vi "GDSProject_GetAllClasses.vi"(1 "AnyProjectItemRefnum":refnum<vi>, 2 "TreeControlRef":refnum<vi>, 3 "ClassProviderName":string, 4 "RootParentTag":string="LabVIEW Object", 5 "error In":errorcluster) -> (15 "ClassPaths":path[](array[path]), 16 "ClassTags":string[](array[string]), 19 "error out":errorcluster)   [LabVIEW 2012]
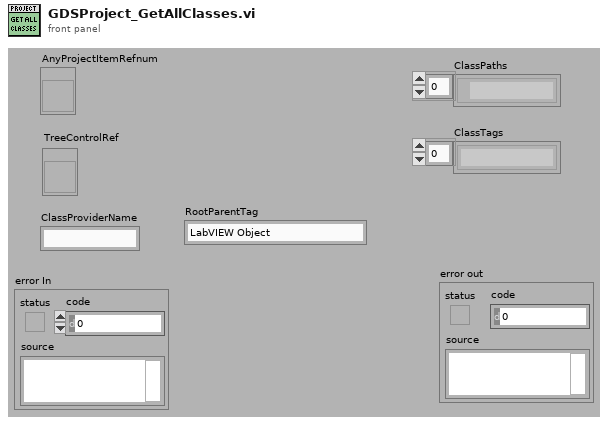
[diagram p1: front panel]
types:
  T1 = cluster{"Classes":refnum<vi>[], "Parents":refnum<vi>[], "ClassIneritance":cluster{string[]}[], "ClassTags":string[], "ClassPaths":path[], "ClassNames":string[]}
  T2 = typedef "GDSLvCLass_ClassSettingsType.ctl" = cluster{"ClassProviderName":string, "ClassTemplateUsed":string, "ClassTemplateVersion":string, "ClassDescription":string, "PlugIns":T3[], "ConnectorPanePattern":string}
  T3 = typedef "GDSLvClass_PlugIn.ctl" = cluster{"Type":T4, "ID":string, "Version":string, "Path":path, "Name":string, "Data":variant}
  T4 = typedef "GDSLvClass_PlugInTypes.ctl" = enum16{"DesignPattern", "MethodTypes"}
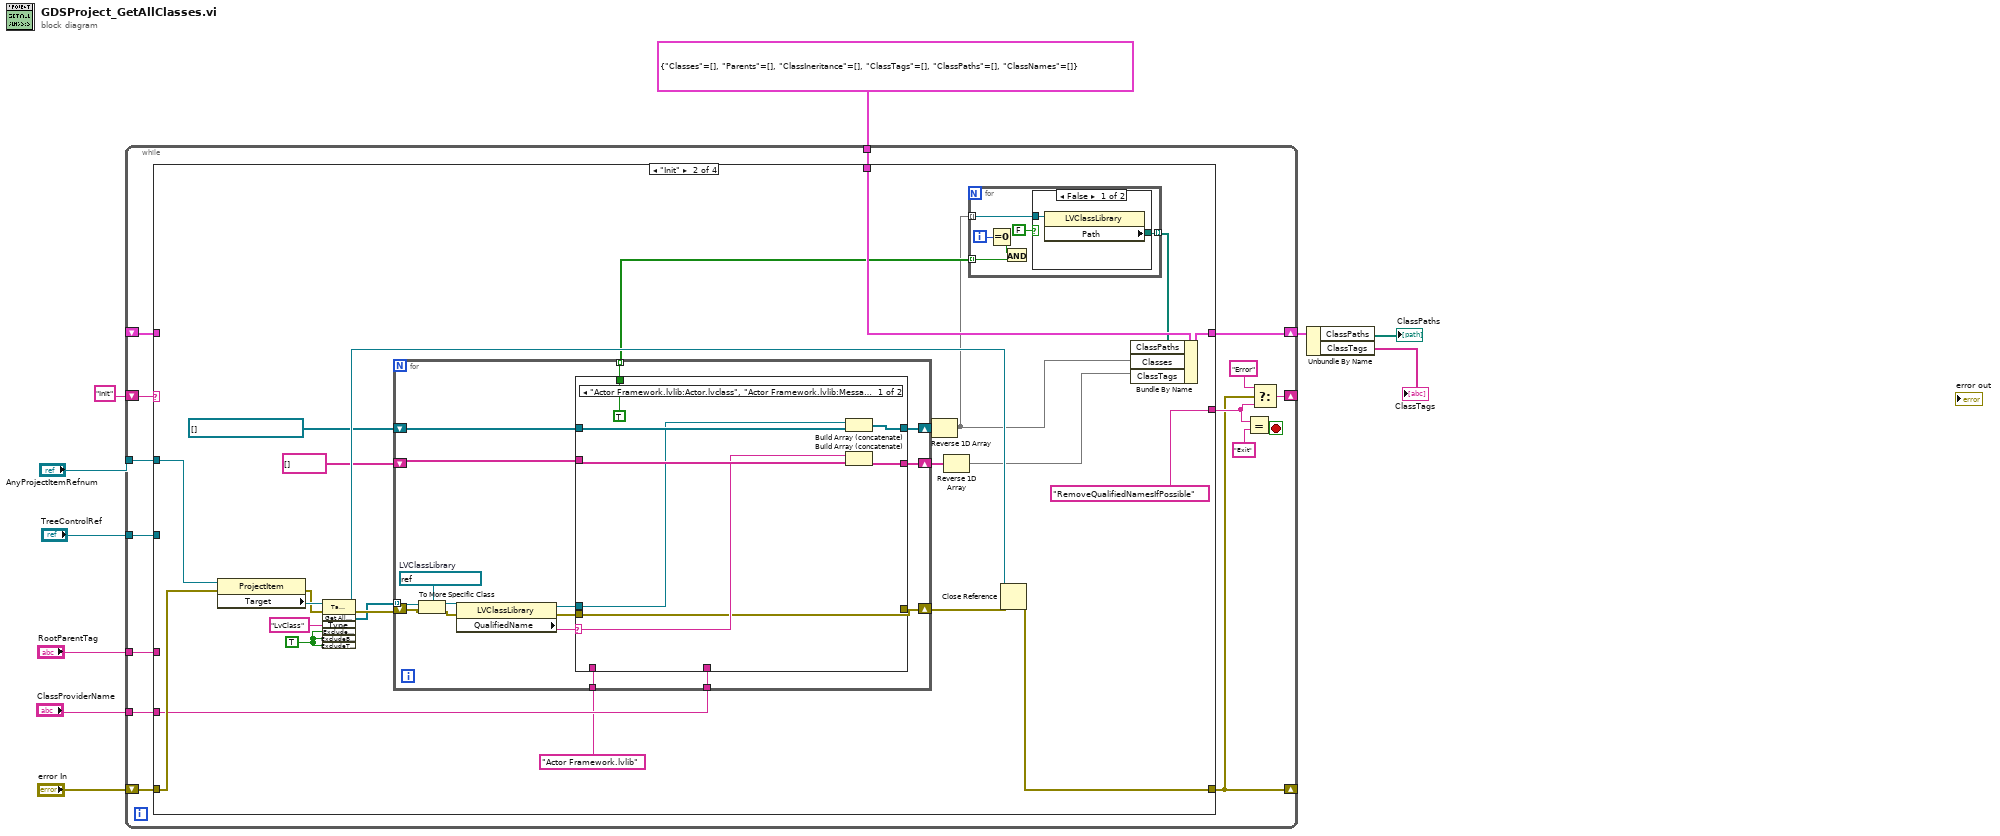
[diagram p0: block diagram]
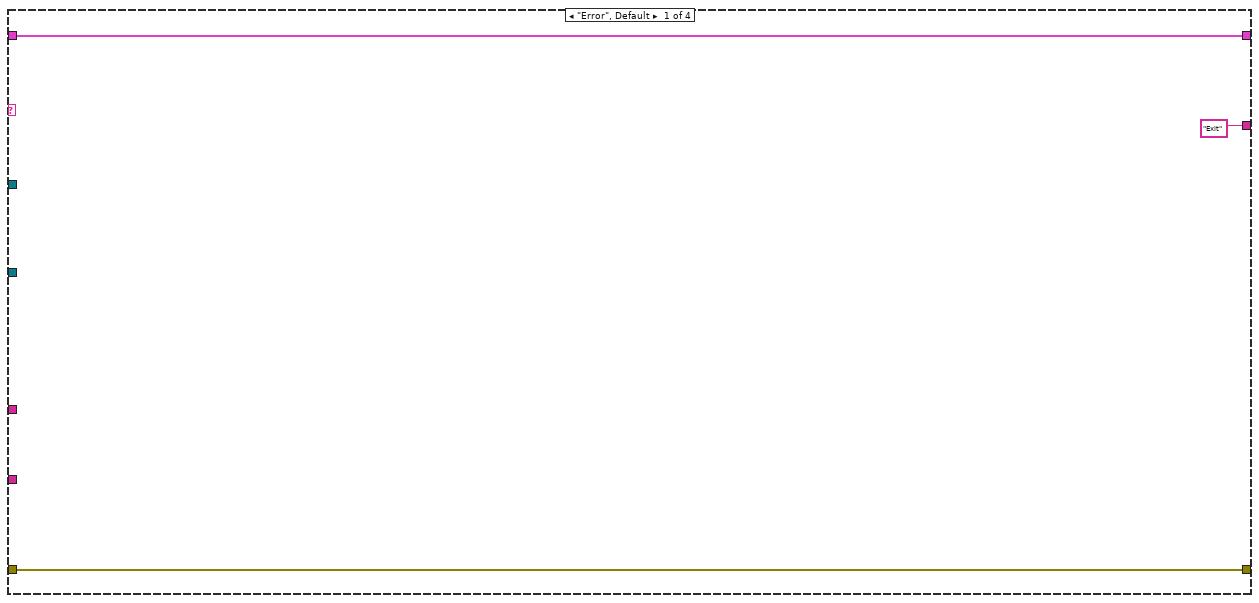
[diagram p2: hidden frame]
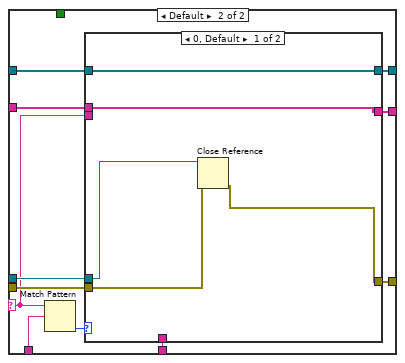
[diagram p4: hidden frame]
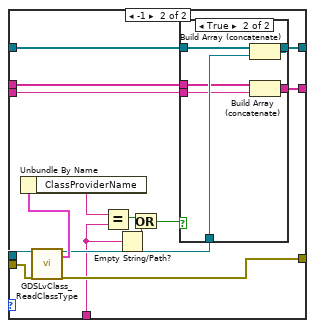
[diagram p5: hidden frame]
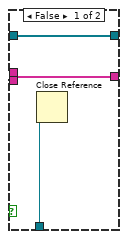
[diagram p6: hidden frame]
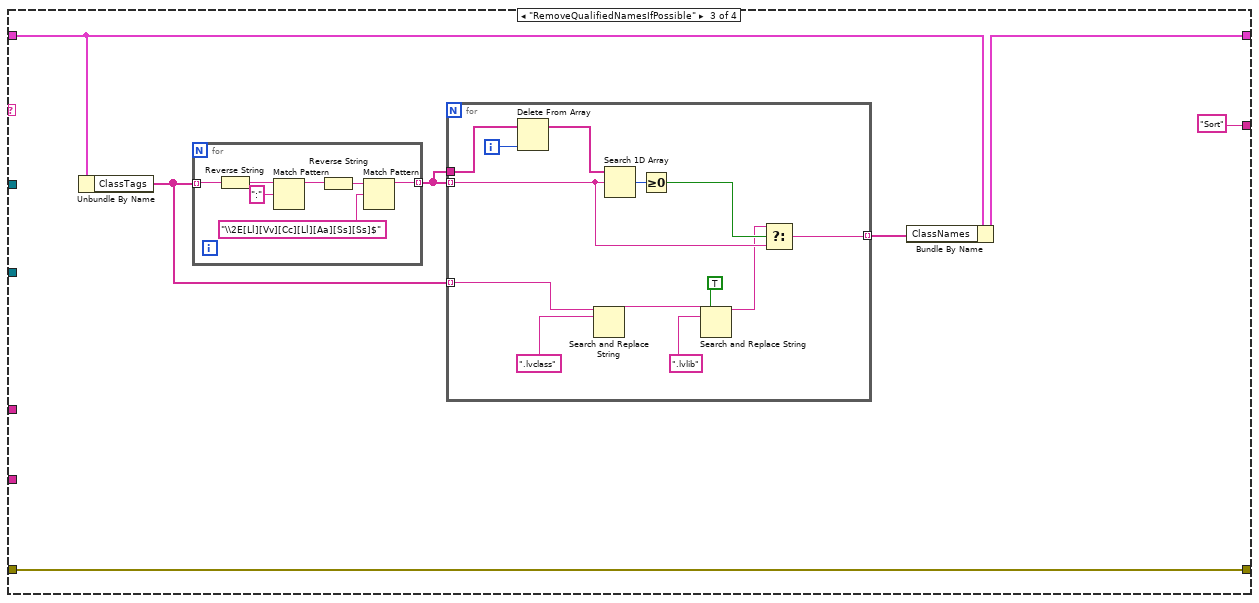
[diagram p7: hidden frame]
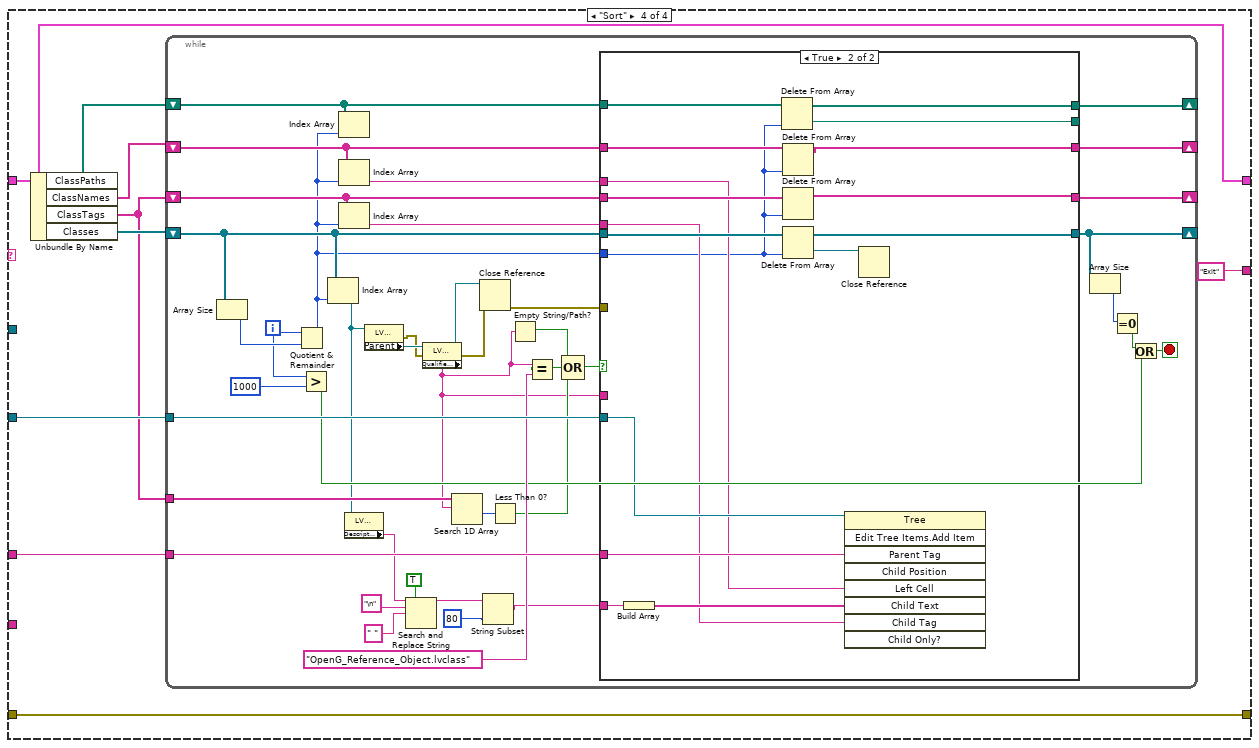
[diagram p8: hidden frame]
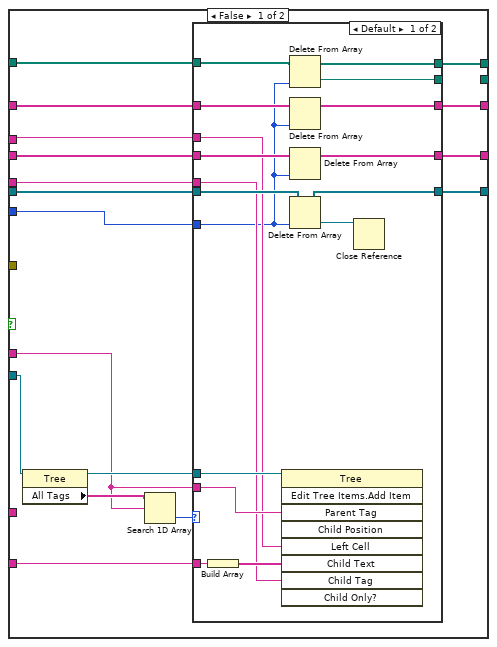
[diagram p9: hidden frame]
diagram:
  n1 = while {
    shift-right: [w18] -> _
    shift-left: "error In" -> [w25]
    shift-right: [w23] -> _
    shift-left: "Init" -> [w24]
    shift-right: [w17] -> w3
    shift-left: _ -> [w16]
    tunnel: "AnyProjectItemRefnum" -> [w15]
    tunnel: T1 {"Classes"=[], "Parents"=[], "ClassIneritance"=[], "ClassTags"=[], "ClassPaths"=[], "ClassNames"=[]} -> [w14]
    tunnel: "ClassProviderName" -> [w13]
    tunnel: "TreeControlRef" -> [w12]
    tunnel: "RootParentTag" -> [w11]
    stop <- w22 stop-if-true
    n2 = case shown="\"Init\"" w24 {
      tunnel: w25 -> [w28 w46 w125 w157]
      tunnel: [w28 w45 w125 w157] -> w18
      tunnel: ["Exit" "RemoveQualifiedNamesIfPossible" "Sort" "Exit"] -> w19
      tunnel: [w26 w43 w127 w155] -> w17
      tunnel: w16 -> [w26 _ w129 w155]
      tunnel: w15 -> [_ w48 _ _]
      tunnel: w14 -> [_ w44 _ _]
      tunnel: w13 -> [_ w42 _ _]
      tunnel: w12 -> [_ _ _ w156]
      tunnel: w11 -> [_ _ _ w158]
      frame "Error", Default {
      }
      frame "Init" {
        w50 = TRUE ("ExcludeDependencies")
        n3 = property class="ProjectItem"(reference=w48, error in=w46) -> (error out=w35:errorcluster, "Target"=w36:refnum<vi>)  [unwired: 1 out]
        n4 = invoke class="TargetItem" method="Get All Descendents"(reference=w36, error in=w35, "Type"="LvClass", "Exclude Dependencies"=w50, "ExcludeBuilds"=w50, "ExcludeTargets"=w50) -> (reference out=w49:refnum<vi>, error out=w47:errorcluster, "All Descendents"=w33:refnum<vi>[])  [unwired: 1 in, 4 out]
        n5 = for {
          tunnel: w33 -> [w76] mode=indexing
          shift-right: [w61] -> w38
          shift-left: refnum<vi>[] [] -> [w74]
          shift-right: [w72] -> w34
          shift-left: w47 -> [w73]
          tunnel: w42 -> [w71]
          shift-right: [w70] -> w39
          shift-left: string[] [] -> [w69]
          tunnel: [w63] -> w32 mode=indexing
          tunnel: "Actor Framework.lvlib" ("Type") -> [w62]
          w75 = refnum<vi> refnum  # LVClassLibrary
          n6 = To More Specific Class(target class=w75, reference=w76, error in=w73) -> (specific class reference=w68:refnum<vi>, error out=w66:errorcluster)
          n7 = property class="LVClassLibrary"(reference=w68, error in=w66) -> (reference out=w67:refnum<vi>, error out=w65:errorcluster, "QualifiedName"=w64:string)
          n8 = case shown="\"Actor Framework.lvlib:Actor.lvclass\", \"Actor Framework.lvlib:Message.lvclass\"" w64 {
            selector: w64 -> [w80 w85]
            tunnel: [w84 w86] -> w61
            tunnel: w74 -> [w78 w95]
            tunnel: [w79 w94] -> w72
            tunnel: w71 -> [_ w93]
            tunnel: [w83 w92] -> w70
            tunnel: w69 -> [w82 w91]
            tunnel: w67 -> [w77 w90]
            tunnel: w65 -> [w79 w89]
            tunnel: [TRUE _] -> w63
            tunnel: w62 -> [_ w88]
            frame "Actor Framework.lvlib:Actor.lvclass", "Actor Framework.lvlib:Message.lvclass" {
              n9 = Build Array (concatenate)(w77, w78) -> (w84:refnum<vi>[])
              n10 = Build Array (concatenate)(w80, w82) -> (w83:string[])
            }
            frame Default {
              n11 = Match Pattern(string=w85, regular expression=w88) -> (offset past match=w87:i32)  [unwired: 1 in, 3 out]
              n12 = case shown="0, Default" w87 {
                tunnel: [w100 w115] -> w86
                tunnel: w95 -> [w100 w114]
                tunnel: [w96 w111] -> w94
                tunnel: w93 -> [_ w109]
                tunnel: [w99 w105] -> w92
                tunnel: w91 -> [w99 w104]
                tunnel: w90 -> [w98 w103]
                tunnel: w89 -> [w97 w102]
                tunnel: w85 -> [_ w101]
                frame 0, Default {
                  n13 = Close Reference(reference=w98, error in (no error)=w97) -> (error out=w96:errorcluster)
                }
                frame -1 {
                  n14 = call <resource>:"GDSLvClass_ReadClassType.vi"("Class Refnum In"=w103, "error in (no error)"=w102) -> ("Class Refnum Out"=w112:refnum<vi>, "ClassSettings"=w113:T2, "error out"=w111:errorcluster)  [unwired: 15 in]
                  n15 = Unbundle By Name(w113) -> ("ClassProviderName"=w110:string)
                  n16 = Equal?(x=w110, y=w109) -> (x = y?=w108:bool)
                  n17 = Empty String/Path?(string/path=w109) -> (empty?=w107:bool)
                  n18 = Or(x=w108, y=w107) -> (x .or. y?=w106:bool)
                  n19 = case shown="True" w106 {
                    tunnel: [w118 w124] -> w115
                    tunnel: w114 -> [w118 w123]
                    tunnel: w112 -> [w117 w122]
                    tunnel: [w116 w121] -> w105
                    tunnel: w104 -> [w116 w120]
                    tunnel: w101 -> [_ w119]
                    frame False {
                      n20 = Close Reference(reference=w117) -> ()  [unwired: 1 in, 1 out]
                    }
                    frame True {
                      n21 = Build Array (concatenate)(w123, w122) -> (w124:refnum<vi>[])
                      n22 = Build Array (concatenate)(w120, w119) -> (w121:string[])
                    }
                  }
                }
              }
            }
          }
        }
        n23 = Reverse 1D Array(array=w38) -> (reversed array=w31:refnum<vi>[])
        n24 = Reverse 1D Array(array=w39) -> (reversed array=w30:string[])
        n25 = for {
          tunnel: w31 -> [w58] mode=indexing
          tunnel: [w57] -> w37 mode=indexing
          tunnel: w32 -> [w54] mode=indexing
          i -> [w56]
          n26 = Equal To 0?(x=w56) -> (x = 0?=w55:bool)
          n27 = And(x=w55, y=w54) -> ()  [unwired: 1 out]
          n28 = case shown="False" FALSE {
            tunnel: w58 -> [w60 _]
            tunnel: [w59 _] -> w57
            frame False {
              n29 = property class="LVClassLibrary"(reference=w60) -> ("Path"=w59:path)  [unwired: 1 in, 2 out]
            }
            frame True {
            }
          }
        }
        n30 = Close Reference(reference=w49, error in (no error)=w34) -> (error out=w45:errorcluster)
        n31 = Bundle By Name(cluster=w44, "ClassPaths"=w37, "Classes"=w31, "ClassTags"=w30) -> (w43:T1)
      }
      frame "RemoveQualifiedNamesIfPossible" {
        n32 = Unbundle By Name(w129) -> ("ClassTags"=w130:string[])
        n33 = for {
          tunnel: w130 -> [w151] mode=indexing
          tunnel: [w145] -> w131 mode=indexing
          n34 = Reverse String(1:w151) -> (0:w150:string)
          n35 = Match Pattern(string=w150, regular expression=":") -> (before substring=w148:string)  [unwired: 1 in, 3 out]
          n36 = Reverse String(1:w148) -> (0:w146:string)
          n37 = Match Pattern(string=w146, regular expression="\\2E[Ll][Vv][Cc][Ll][Aa][Ss][Ss]$") -> (before substring=w145:string)  [unwired: 1 in, 3 out]
        }
        n38 = for {
          tunnel: w131 -> [w142] mode=indexing
          tunnel: w131 -> [w140]
          tunnel: w130 -> [w133] mode=indexing
          tunnel: [w141] -> w128 mode=indexing
          i -> [w138]
          n39 = Delete From Array(array=w140, index=w138) -> (array with subset deleted=w139:string[])  [unwired: 1 in, 1 out]
          n40 = Search and Replace String(input string=w133, search string=".lvclass" ("regular expression")) -> (result string=w134:string)  [unwired: 6 in, 3 out]
          n41 = Search 1D Array(1D array=w139, element=w142) -> (index of element=w144:i32)  [unwired: 1 in]
          n42 = Greater Or Equal To 0?(x=w144) -> (x >= 0?=w143:bool)
          n43 = Search and Replace String(replace all?=TRUE ("replace all? (F)"), input string=w134, search string=".lvlib" ("regular expression")) -> (result string=w135:string)  [unwired: 5 in, 3 out]
          n44 = Select(t=w135, s=w143, f=w142) -> (s? t:f=w141:string)
        }
        n45 = Bundle By Name(cluster=w129, "ClassNames"=w128) -> (w127:T1)
      }
      frame "Sort" {
        n46 = Unbundle By Name(w155) -> ("ClassPaths"=w152:path[], "ClassNames"=w154:string[], "ClassTags"=w153:string[], "Classes"=w160:refnum<vi>[])
        n47 = while {
          shift-right: [w199] -> _
          shift-left: w160 -> [w200]
          tunnel: w156 -> [w201]
          tunnel: w158 -> [w196]
          tunnel: w153 -> [w186]
          shift-right: [w177] -> _
          shift-left: w153 -> [w176]
          shift-right: [w173] -> _
          shift-left: w154 -> [w174]
          shift-right: [w161] -> _
          shift-left: w152 -> [w162]
          i -> [w189]
          stop <- w190 stop-if-true
          n48 = Array Size(array=w200) -> (size(s)=w197:i32)
          n49 = Quotient & Remainder(x=w189, y=w197) -> (x-y*floor(x/y)=w163:i32)  [unwired: 1 out]
          n50 = Greater?(x=w189, y=1000) -> (0:w187:bool)
          n51 = Index Array(array=w200, index=w163) -> (element=w170:refnum<vi>)
          n52 = Index Array(array=w162, index=w163) -> ()  [unwired: 1 out]
          n53 = Index Array(array=w174, index=w163) -> (element=w171:string)
          n54 = Index Array(array=w176, index=w163) -> (element=w175:string)
          n55 = property class="LVClassLibrary"(reference=w170) -> ("Description"=w172:string)  [unwired: 1 in, 2 out]
          n56 = property class="LVClassLibrary"(reference=w170) -> (error out=w167:errorcluster, "Parent"=w178:refnum<vi>)  [unwired: 1 in, 1 out]
          n57 = Search and Replace String(replace all?=TRUE ("replace all? (F)"), input string=w172, search string="\n" ("replace string (\"\")"), replace string=" " ("replace string (\"\")")) -> (result string=w182:string)  [unwired: 4 in, 3 out]
          n58 = property class="LVClassLibrary"(reference=w178, error in=w167) -> (reference out=w169:refnum<vi>, error out=w168:errorcluster, "QualifiedName"=w165:string)
          n59 = Search 1D Array(1D array=w186, element=w165) -> (index of element=w185:i32)  [unwired: 1 in]
          n60 = Close Reference(reference=w169, error in (no error)=w168) -> (error out=w166:errorcluster)
          n61 = String Subset(string=w182, length (rest)=80 ("length (rest)")) -> (substring=w180:string)  [unwired: 1 in]
          n62 = Less Than 0?(x=w185) -> (x < 0?=w184:bool)
          n63 = Empty String/Path?(string/path=w165) -> (empty?=w195:bool)
          n64 = Equal?(x=w165, y="OpenG_Reference_Object.lvclass") -> (x = y?=w193:bool)
          n65 = Compound Arithmetic op=OR(w195, w193, w184) -> (w194:bool)
          n66 = case shown="True" w194 {
            tunnel: w201 -> [w218 w256]
            tunnel: w200 -> [w214 w255]
            tunnel: w163 -> [w213 w242]
            tunnel: [w212 w254] -> w199
            tunnel: w180 -> [w211 w246]
            tunnel: w196 -> [_ w251]
            tunnel: w176 -> [w210 w250]
            tunnel: [w209 w249] -> w177
            tunnel: w175 -> [w208 w245]
            tunnel: w174 -> [w207 w248]
            tunnel: [w206 w247] -> w173
            tunnel: w171 -> [w205 w244]
            tunnel: w165 -> [w204 _]
            tunnel: w166 -> [_ _]
            tunnel: w162 -> [w203 w243]
            tunnel: [w202 w241] -> w161
            tunnel: [_ w240] -> _
            frame False {
              n67 = property class="Tree"(reference=w218) -> (reference out=w215:refnum<vi>, "All Tags"=w217:string[])  [unwired: 1 in, 1 out]
              n68 = Search 1D Array(1D array=w217, element=w204) -> (index of element=w216:i32)  [unwired: 1 in]
              n69 = case shown="Default" w216 {
                tunnel: w215 -> [w235 _]
                tunnel: w204 -> [w234 _]
                tunnel: w214 -> [w233 w239]
                tunnel: w213 -> [w220 _]
                tunnel: [w232 w239] -> w212
                tunnel: w211 -> [w230 _]
                tunnel: w210 -> [w228 w238]
                tunnel: [w227 w238] -> w209
                tunnel: w208 -> [w226 _]
                tunnel: w207 -> [w225 w237]
                tunnel: [w224 w237] -> w206
                tunnel: w205 -> [w223 _]
                tunnel: w203 -> [w222 w236]
                tunnel: [w221 w236] -> w202
                tunnel: [w219 _] -> _
                frame Default {
                  n70 = Build Array(w230) -> (w229:string[])
                  n71 = invoke class="Tree" method="Edit Tree Items.Add Item"(reference=w235, "Parent Tag"=w234, "Left Cell"=w223, "Child Text"=w229, "Child Tag"=w226) -> ()  [unwired: 4 in, 9 out]
                  n72 = Delete From Array(array=w222, index=w220) -> (deleted portion=w219:path, array with subset deleted=w221:path[])  [unwired: 1 in]
                  n73 = Delete From Array(array=w225, index=w220) -> (array with subset deleted=w224:string[])  [unwired: 1 in, 1 out]
                  n74 = Delete From Array(array=w228, index=w220) -> (array with subset deleted=w227:string[])  [unwired: 1 in, 1 out]
                  n75 = Delete From Array(array=w233, index=w220) -> (deleted portion=w231:refnum<vi>, array with subset deleted=w232:refnum<vi>[])  [unwired: 1 in]
                  n76 = Close Reference(reference=w231) -> ()  [unwired: 1 in, 1 out]
                }
                frame -1 {
                }
              }
            }
            frame True {
              n77 = Build Array(w246) -> (w252:string[])
              n78 = Delete From Array(array=w243, index=w242) -> (deleted portion=w240:path, array with subset deleted=w241:path[])  [unwired: 1 in]
              n79 = Delete From Array(array=w248, index=w242) -> (array with subset deleted=w247:string[])  [unwired: 1 in, 1 out]
              n80 = Delete From Array(array=w250, index=w242) -> (array with subset deleted=w249:string[])  [unwired: 1 in, 1 out]
              n81 = Delete From Array(array=w255, index=w242) -> (deleted portion=w253:refnum<vi>, array with subset deleted=w254:refnum<vi>[])  [unwired: 1 in]
              n82 = invoke class="Tree" method="Edit Tree Items.Add Item"(reference=w256, "Parent Tag"=w251, "Left Cell"=w244, "Child Text"=w252, "Child Tag"=w245) -> ()  [unwired: 4 in, 9 out]
              n83 = Close Reference(reference=w253) -> ()  [unwired: 1 in, 1 out]
            }
          }
          n84 = Array Size(array=w199) -> (size(s)=w198:i32)
          n85 = Equal To 0?(x=w198) -> (x = 0?=w191:bool)
          n86 = Or(x=w191, y=w187) -> (x .or. y?=w190:bool)
        }
      }
    }
    n87 = Equal?(x=w19, y="Exit") -> (x = y?=w22:bool)
    n88 = Select(t="Error", s=w18, f=w19) -> (s? t:f=w23:string)
  }
  n89 = Unbundle By Name(w3) -> ("ClassPaths"=→"ClassPaths":path[], "ClassTags"=→"ClassTags":string[])
